vi "rSetup.vi"(0 "Socket in":refnum<class "Socket.lvclass">, 11 "error in (no error)":errorcluster) -> (4 "Socket out":refnum<class "Socket.lvclass">, 6 "IP Address":string, 8 "Port":u16, 15 "error out":errorcluster)   [LabVIEW 2011, in "Socket.lvclass"]
uses:
  Socket.lvclass
  Socket.lvclass/Socket.ctl
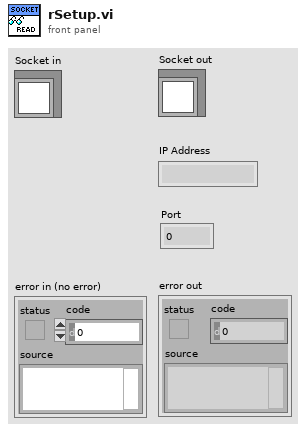
[diagram p1: front panel]
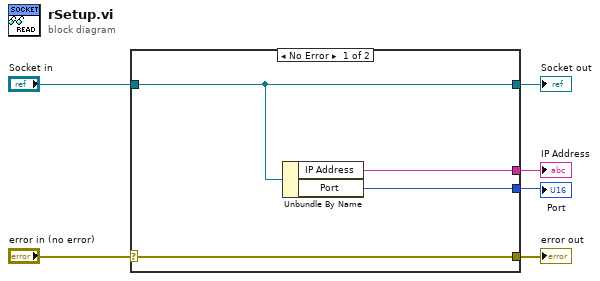
[diagram p0: block diagram]
diagram:
  n1 = case shown="No Error" "error in (no error)" {
    selector: "error in (no error)" -> [w10 w11]
    tunnel: [w10 w11] -> w5
    tunnel: [w9 w12] -> w3
    tunnel: "Socket in" -> [w9 w12]
    tunnel: [w8 _] -> w2
    tunnel: [w7 _] -> w1
    frame No Error {
      n2 = Unbundle By Name(w9) -> ("IP Address"=w8:string, "Port"=w7:u16)
    }
    frame Error {
    }
  }
  "error out" <- w5
  "Socket out" <- w3
  "IP Address" <- w2
  "Port" <- w1
